vi "Read Dependencies.vi"(8 "error in (no error)":errorcluster, 11 "Transport in":refnum<class "Transport.lvclass">) -> (0 "error out":errorcluster, 2 "Dependencies":T1, 3 "Transport out":refnum<class "Transport.lvclass">)   [LabVIEW 2016, in "Transport.lvclass"]
uses:
  Transport.lvclass
  Typedefs/Dependencies--Cluster.ctl
  SweepControl/SweepControl.lvclass
  Transport.lvclass/Transport.ctl
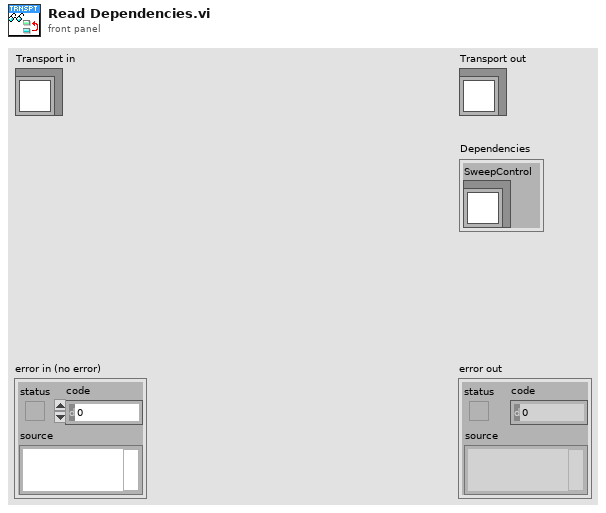
[diagram p1: front panel]
types:
  T1 = typedef "Transport.lvclass/Dependencies--Cluster.ctl" = cluster{"SweepControl":refnum<class "SweepControl.lvclass">}
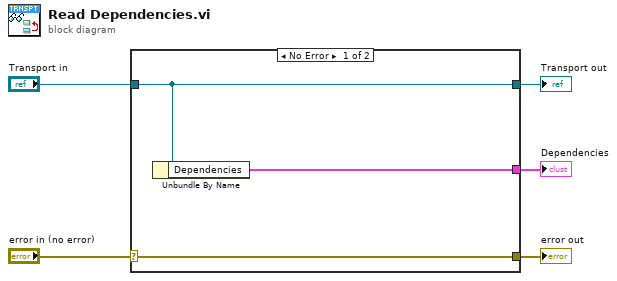
[diagram p0: block diagram]
diagram:
  n1 = case shown="No Error" "error in (no error)" {
    selector: "error in (no error)" -> [w8 w9]
    tunnel: [w8 w9] -> w4
    tunnel: [w7 w10] -> w2
    tunnel: "Transport in" -> [w7 w10]
    tunnel: [w6 _] -> w1
    frame No Error {
      n2 = Unbundle By Name(w7) -> ("Dependencies"=w6:T1)
    }
    frame Error {
    }
  }
  "error out" <- w4
  "Transport out" <- w2
  "Dependencies" <- w1
